vi "Queue_Processing.vi"(6 "Delay(ms)":u32, 7 "loop val":i32=1, 8 "error in (no error)":errorcluster caption="错误输入（无错误）", 9 "Data Array":variant[](array[variant]), 10 "Cmd Array":string[](array[string]), 11 "Call Array":string[](array[string])=["CAN_Demo0", "LIN_Demo0"]) -> (0 "error out":errorcluster caption="错误输出")   [LabVIEW 2014]
uses:
  <vilib>/Utility/miscctls.llb/LVPointTypeDef.ctl
panel:
  out "Processing...":u8(slide) scale=0.0..100.0
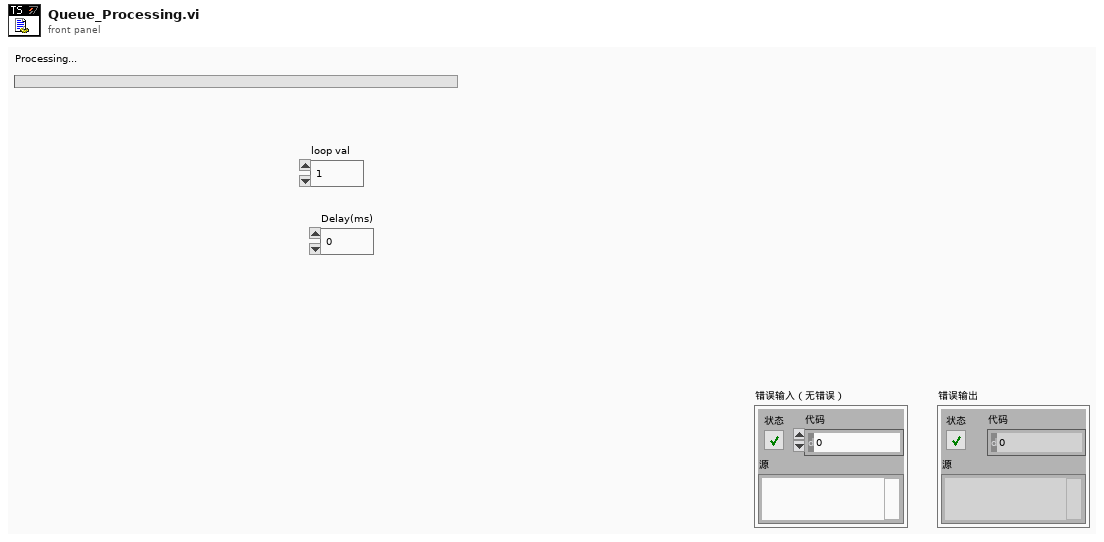
[diagram p1: front panel]
types:
  T1 = typedef "LVPointTypeDef.ctl" = cluster{"Horizontal":i16, "Vertical":i16}
  T2 = cluster{"Sender":string, "receiver":string, "message":string, "data":variant}
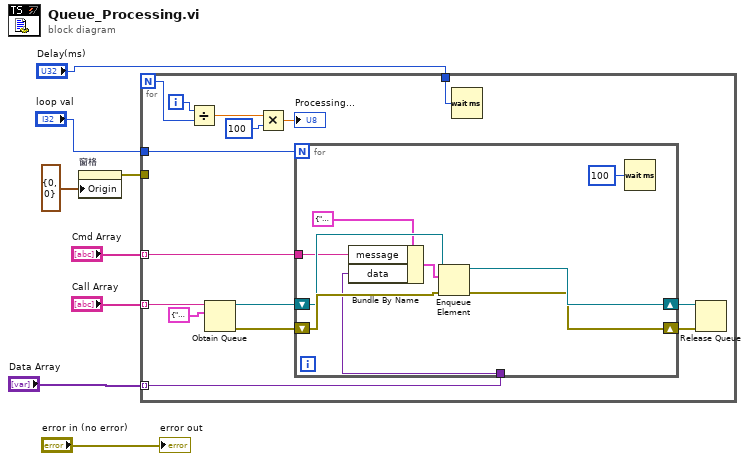
[diagram p0: block diagram]
diagram:
  n1 = property on="窗格" class="Pane"("Origin"=T1 {"Horizontal"=0, "Vertical"=0} ("原点")) -> (error out=w7:errorcluster)  [unwired: 2 in, 1 out]
  n2 = for {
    N -> [w13]
    tunnel: "Call Array" -> [w19] mode=indexing
    tunnel: w7 -> [_]
    tunnel: "Cmd Array" -> [w12] mode=indexing
    tunnel: "Data Array" -> [w11] mode=indexing
    tunnel: "Delay(ms)" -> [w10]
    tunnel: "loop val" -> [w9]
    i -> [w14]
    n3 = Divide(x=w14, y=w13) -> (x/y=w17:dbl)
    n4 = Obtain Queue(name (unnamed)=w19, element data type=T2 {"Sender"="", "receiver"="", "message"="", "data"=variant} ("Communication message")) -> (queue out=w23:refnum<queue>, error out=w21:errorcluster)  [unwired: 3 in, 1 out]
    n5 = Multiply(x=w17, y=u8 100) -> (x*y=→"Processing...":dbl)
    n6 = for {
      N: w9 -> [_]
      shift-right: [w32] -> w22
      shift-left: w23 -> [w29]
      shift-right: [w31] -> w20
      shift-left: w21 -> [w30]
      tunnel: w12 -> [w28]
      tunnel: w11 -> [w27]
      n7 = Bundle By Name(cluster=T2 {"Sender"="", "receiver"="", "message"="Quit", "data"=variant} ("元素"), "message"=w28, "data"=w27) -> (w24:T2)
      n8 = Enqueue Element(queue=w29, element=w24, error in (no error)=w30) -> (queue out=w32:refnum<queue>, error out=w31:errorcluster)  [unwired: 1 in, 1 out]
      n9 = Wait (ms)(milliseconds to wait=u32 100 ("等待时间（毫秒）")) -> ()  [unwired: 1 out]
    }
    n10 = Wait (ms)(milliseconds to wait=w10) -> ()  [unwired: 1 out]
    n11 = Release Queue(queue=w22, error in (no error)=w20) -> ()  [unwired: 1 in, 3 out]
  }
  "error out" <- "error in (no error)"
